vi "UpdateUserInterface.vi"(8 "error in (no error)":errorcluster, 10 "DataExchange":T1, 11 "DisplayerUI in":refnum<class "DisplayerUI.lvclass">) -> (0 "error out":errorcluster, 2 "DataExchange Out":T1, 3 "DisplayerUI out":refnum<class "DisplayerUI.lvclass">)   [LabVIEW 2020, in "DisplayerUI.lvlib" / "DisplayerUI.lvclass"]
uses:
  DisplayerUI.lvclass
  Hardware Abstraction Layer/Component/Device/Device/DataExchange.ctl
  DisplayerUI.lvclass/DisplayerUI.ctl
  <vilib>/vision/Image Controls.llb/IMAQ Image.ctl
  Hardware Abstraction Layer/Component/GenericActor/GenericActor/GenericController.lvclass
  Interface/DataListener/DataListener.lvclass
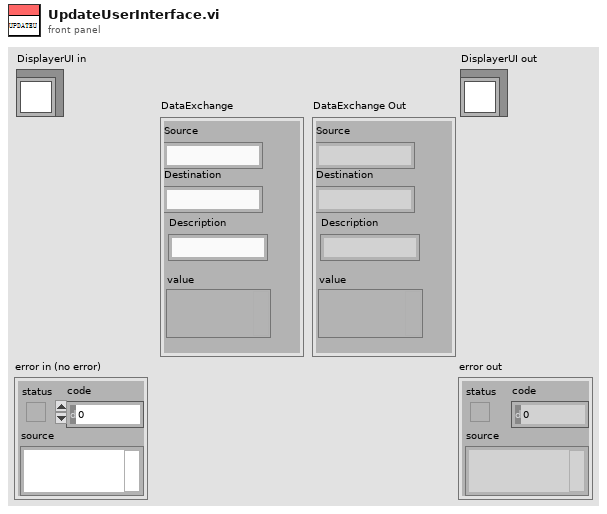
[diagram p1: front panel]
types:
  T1 = typedef "DataListener.lvclass/DataExchange.ctl" = cluster{"Source":string, "Destination":string, "Description":string, "value":variant}
  T2 = typedef "IMAQ Image.ctl" = refnum<image>
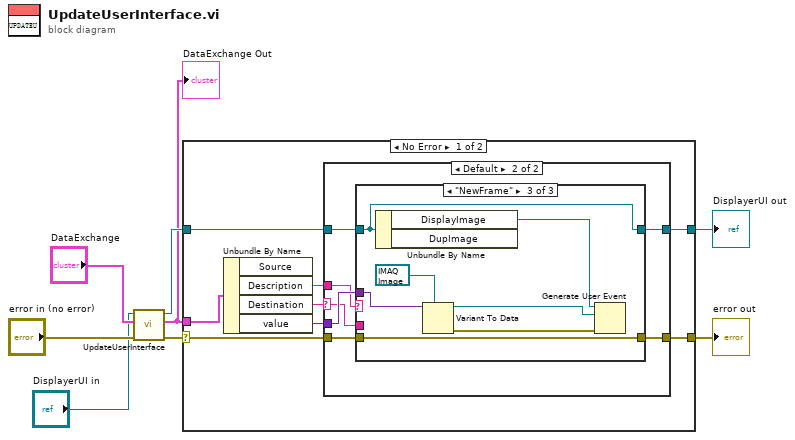
[diagram p0: block diagram]
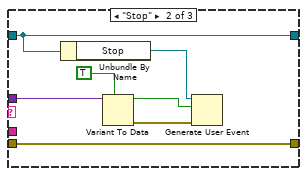
[diagram p4: hidden frame]
diagram:
  n1 = call-parent "UpdateUserInterface.vi"("error in (no error)"="error in (no error)", "DataExchange"="DataExchange", "GenericController in"="DisplayerUI in") -> ("error out"=w4:errorcluster, "DataExchange Out"=w3:T1, "GenericController out"=w5:refnum<class "DisplayerUI.lvclass">)  [unwired: 6 in]
  "DataExchange Out" <- w3
  n2 = case shown="No Error" w4 {
    selector: w4 -> [w11 w43]
    tunnel: [w10 w43] -> w1
    tunnel: [w12 w42] -> w2
    tunnel: w5 -> [w13 w42]
    tunnel: w3 -> [w16 _]
    frame No Error {
      n3 = Unbundle By Name(w16) -> ("Description"=w14:string, "Destination"=w9:string, "value"=w15:variant)  [unwired: 1 out]
      n4 = case shown="Default" w9 {
        selector: w9 -> [_ w19]
        tunnel: w15 -> [_ w25]
        tunnel: w14 -> [_ w24]
        tunnel: w13 -> [w18 w23]
        tunnel: [w18 w22] -> w12
        tunnel: w11 -> [w17 w21]
        tunnel: [w17 w20] -> w10
        frame "duplicate this case" {
        }
        frame Default {
          n5 = case shown="\"NewFrame\"" w24 {
            tunnel: w25 -> [_ w34 w41]
            tunnel: [w27 w29 w38] -> w22
            tunnel: w23 -> [w27 w29 w38]
            tunnel: [w26 w28 w37] -> w20
            tunnel: w21 -> [w26 w28 w37]
            tunnel: w19 -> [_ _ _]
            frame Default {
            }
            frame "Stop" {
              n6 = Unbundle By Name(w29) -> ("Stop"=w33:refnum<user-event>)
              n7 = Variant To Data(type=TRUE, Variant=w34) -> (data=w32:bool, error out=w30:errorcluster)  [unwired: 1 in]
              n8 = Generate User Event(user event=w33, event data cluster=w32, error in=w30) -> ()  [unwired: 1 in, 2 out]
            }
            frame "NewFrame" {
              n9 = Unbundle By Name(w38) -> ("DisplayImage"=w40:refnum<user-event>)  [unwired: 1 out]
              n10 = Variant To Data(type=T2 refnum ("event data"), Variant=w41) -> (data=w35:T2, error out=w39:errorcluster)  [unwired: 1 in]
              n11 = Generate User Event(user event=w40, event data cluster=w35, error in=w39) -> ()  [unwired: 1 in, 2 out]
            }
          }
        }
      }
    }
    frame Error {
    }
  }
  "error out" <- w1
  "DisplayerUI out" <- w2
